vi "gnd_without 3d.vi"() -> ()   [LabVIEW 2015]
doc: "This example performs writes and reads on a serial port, as directed by the user. You can press the Write and Read buttons, and change the Read Count, while the example is running.\n\nThe parameters set for the serial port must match the parameters of the connected instrument or device. In this example, the Read Count parameter specifies the number of bytes that the serial port reads. If there were more bytes at the port than the specified number, those bytes would not be read. If there were less bytes at the port than the specified number, you would receive a timeout error.\n\nThis example expands upon the flow control options for XON and XOFF, allowing the user to choose those control characters. Also, the user can enable or disable a termination character. Some devices require a termination character in order to identify the end of command strings. Some devices send a termination character to signify the end of data to be read. This example shows how you can end the Read operation once a termination character is detected in the buffer and/or append a termination character at the end of the Write data."
uses:
  Program Files/National Instruments/LabVIEW 2015/examples/Instrument IO/Serial/support/Serial - Settings.ctl
  <vilib>/Instr/_visa.llb/VISA Configure Serial Port (Instr).vi
panel:
  out "Euler Angle Chart":cluster{"Pitch":sgl, "Roll":sgl, "Yaw":sgl}(graph)
  out "Servo Angle Chart":T1(graph)
  in  "Period":u32=50
  out "Frequency":dbl
  out "Right_Servo_Angle":string
  out "Left_Servo_Angle":string
  out "Altitude":string
  out "Latitude":string
  in  "Current Satellite Position":refnum<k7>(container)
  out "String":string
  out "current time":timestamp format="%<%H:%M:%S%2u>T"
  out "Longditude":string
  out "Yaw":string
  out "Roll":string
  out "Pitch":string
  out "Start Byte":string
  out "From":string
  in  "Read Count":u32=1000
  in  "Stop Button":bool
  out "length":i32
  out "substring":string
  in  "Start Byte":string
  out "Data Log":string
  in  "Serial Settings":T2={"baud rate"=9600, "data bits"=8, "parity"=enum."None", "stop bits"=10, "flow control"=0} {"flow control" items=["None"=0, "XON/XOFF"=1, "RTS/CTS"=2, "DTR/DSR"=4]; "stop bits" items=["1.0"=10, "1.5"=15, "2.0"=20]; "data bits" min=5 max=8 step=1; "baud rate" items=["75"=75, "110"=110, "134"=134, "150"=150, "300"=300, "600"=600, "1200"=1200, "1800"=1800, "2400"=2400, "4800"=4800, "7200"=7200, "9600"=9600, "14400"=14400, "19200"=19200, "28800"=28800, "38400"=38400, "56000"=56000, "57600"=57600, "115200"=115200, "128000"=128000, "230400"=230400]}
  in  "VISA resource name":refnum<visa-resource-name>="COM1"
  # "2016 SNUSAT CANSAT Competition\nGround Station"
  # "Serial Port Setting"
  # "Serial Read Setting"
  # "Satellite Attitude\n(Euler Angle)"
  # "GPS Position"
  # "Frequency Set (f = 1 / T)"
  # "Servo Angle State"
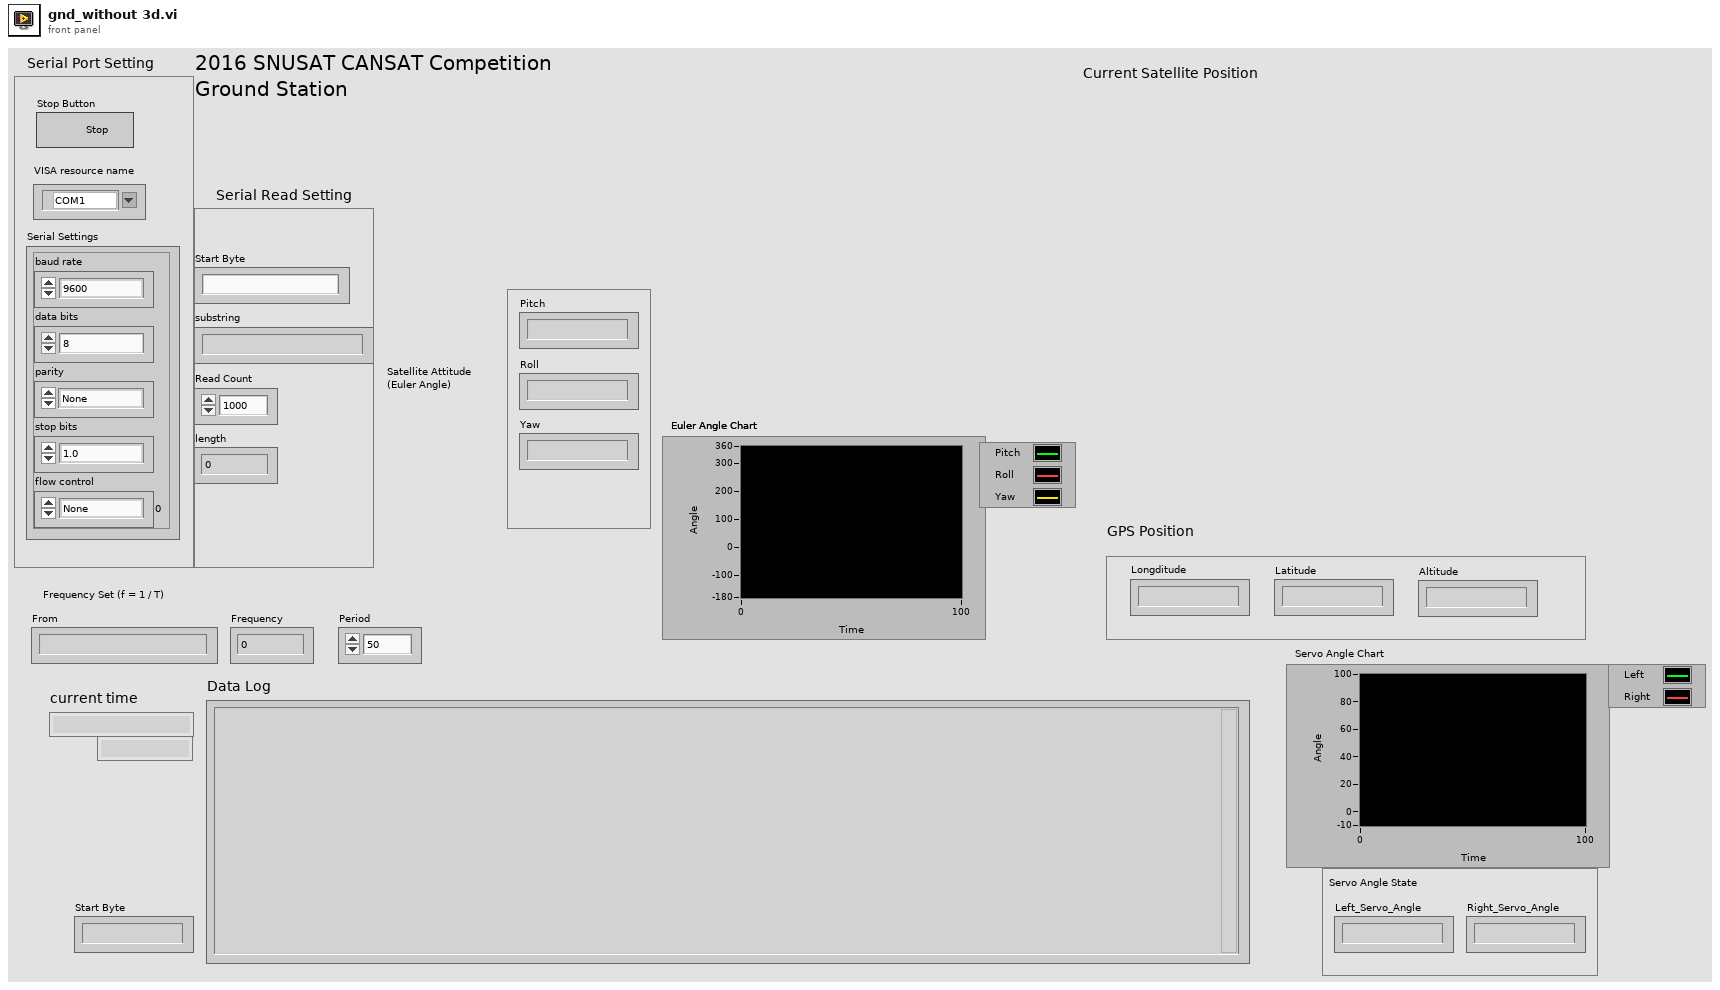
[diagram p1: front panel]
types:
  T1 = cluster{"Left_Servo_Angle":sgl, "Right_Servo_Angle":sgl}
  T2 = typedef "Serial - Settings.ctl" = cluster{"baud rate":u32, "data bits":u16, "parity":enum16{"None", "Odd", "Even", "Mark", "Space"}, "stop bits":u16, "flow control":u16}
  T3 = cluster{"Pitch":string, "Roll":string, "Yaw":string}
  T4 = cluster{"Left_Servo_Angle":string, "Right_Servo_Angle":string}
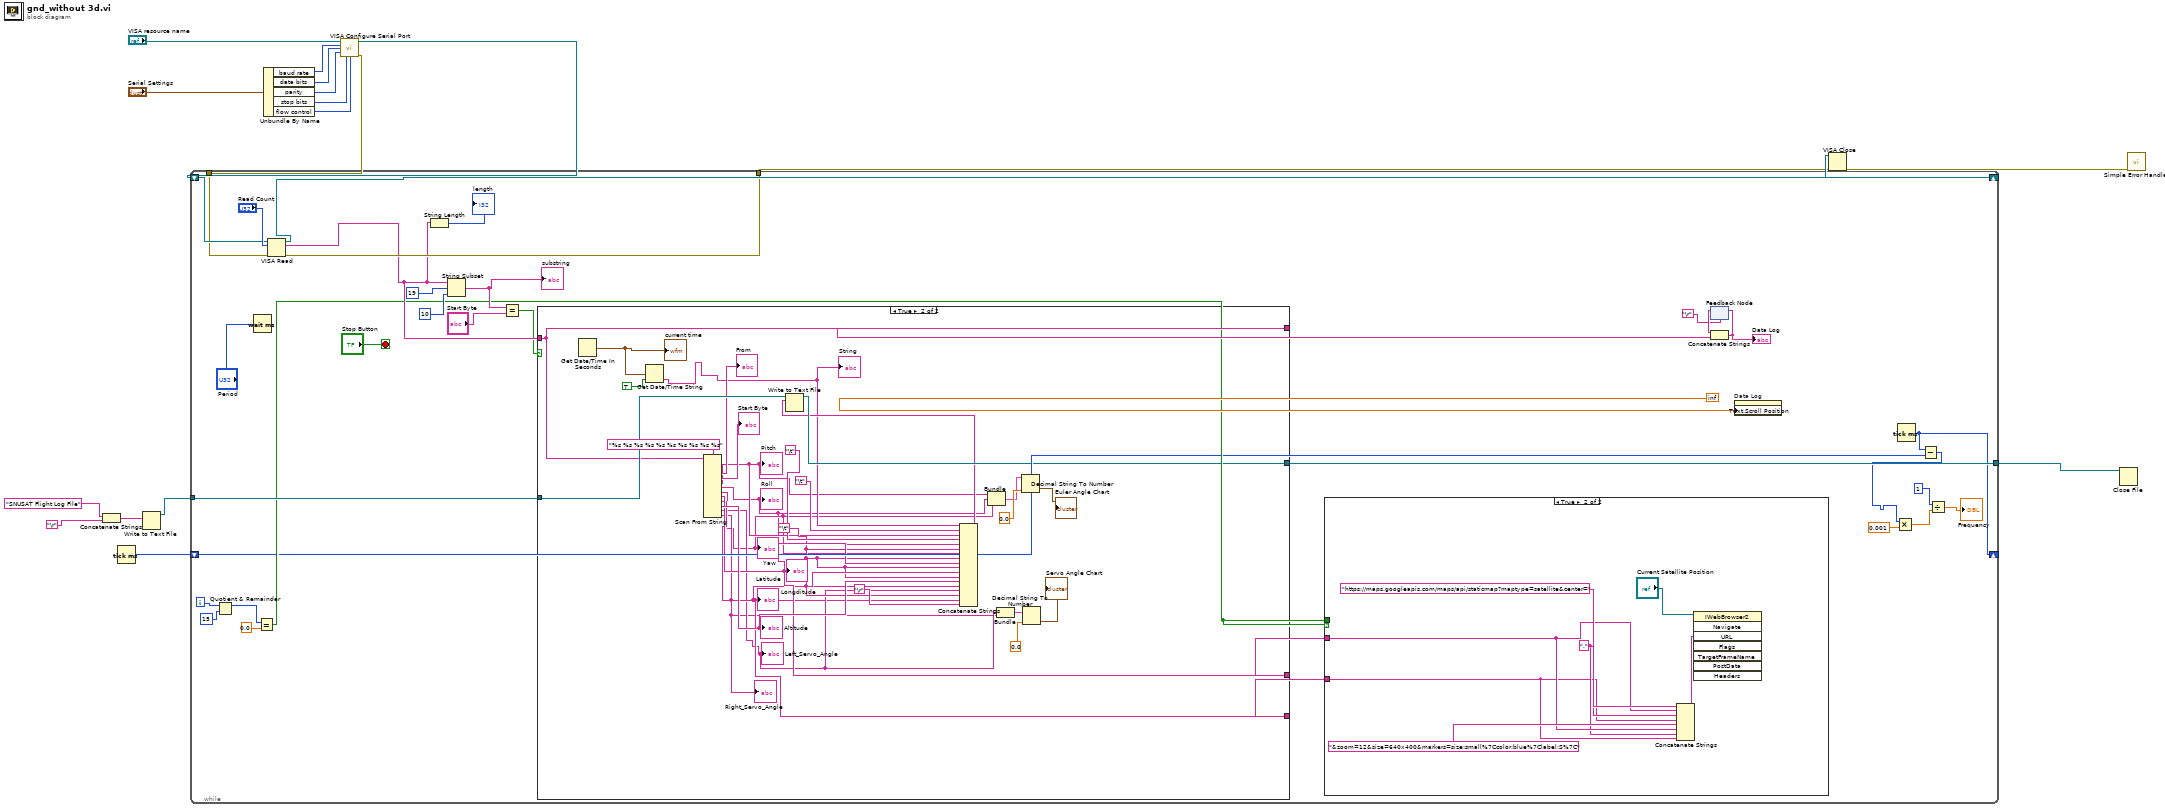
[diagram p0: block diagram]
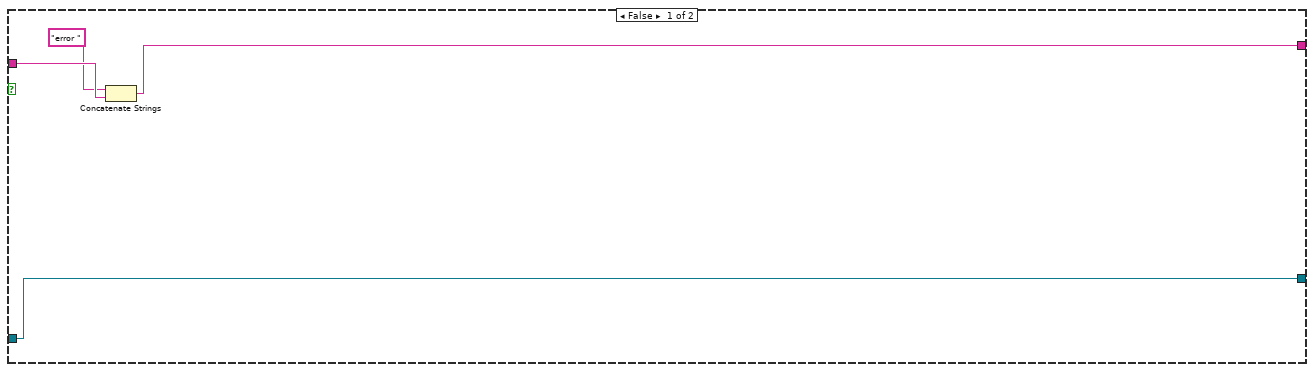
[diagram p3: hidden frame]
diagram:
  n1 = Concatenate Strings("SNUSAT Flight Log File", "\r") -> (w2:string)
  n2 = Tick Count (ms)() -> (millisecond timer value=w1:u32)
  n3 = Write to Text File(text=w2) -> (refnum out=w6:refnum<file>)  [unwired: 3 in, 2 out]
  n4 = Unbundle By Name("Serial Settings") -> ("baud rate"=w14:u32, "data bits"=w15:u16, "parity"=w16:enum16{"None", "Odd", "Even", "Mark", "Space"}, "stop bits"=w17:u16, "flow control"=w11:u16)
  n5 = call-poly "VISA Configure Serial Port"("VISA resource name"="VISA resource name", "baud rate (9600)"=w14, "data bits (8)"=w15, "parity (0:none)"=w16, "stop bits (10: 1 bit)"=w17, "flow control (0:none)"=w11) -> ("VISA resource name out"=w8:refnum<visa-resource-name>, "error out"=w7:errorcluster)  [unwired: 4 in, 4 out]
  n6 = while {
    tunnel: w7 -> [w51]
    tunnel: [w49] -> w9
    shift-right: [w50] -> w10
    shift-left: w8 -> [w52]
    tunnel: w6 -> [w36]
    tunnel: [w35] -> w5
    shift-right: [w19] -> _
    shift-left: w1 -> [w21]
    i -> [w32]
    stop <- "Stop Button" stop-if-true
    n7 = Quotient & Remainder(x=w32, y=15) -> (x-y*floor(x/y)=w29:i32)  [unwired: 1 out]
    n8 = Wait (ms)(milliseconds to wait="Period") -> ()  [unwired: 1 out]
    n9 = Equal?(x=w29, y=0.0) -> (x = y?=w26:bool)
    n10 = VISA Read(VISA resource name=w52, byte count="Read Count", error in (no error)=w51) -> (VISA resource name out=w50:refnum<visa-resource-name>, read buffer=w41:string, error out=w49:errorcluster)  [unwired: 1 out]
    n11 = String Length(string=w41) -> (length=→"length":i32)
    n12 = String Subset(string=w41, offset (0)=19, length (rest)=10 ("length (rest)")) -> (substring=w43:string)
    "substring" <- w43
    n13 = Equal?(x=w43, y="Start Byte") -> (x = y?=w33:bool)
    n14 = case shown="True" w33 {
      tunnel: w41 -> [w64 w87]
      tunnel: [w62 w87] -> w40
      tunnel: w36 -> [w61 w92]
      tunnel: [w61 w91] -> w35
      tunnel: [_ w79] -> w28
      tunnel: [_ w78] -> w27
      frame False {
        n15 = Concatenate Strings("error " ("string"), w64) -> (w62:string)
      }
      frame True {
        w76 = "\t"
        n16 = Get Date/Time In Seconds() -> (seconds since 1Jan1904=w83:timestamp)
        "current time" <- w83
        n17 = Get Date/Time String(seconds (now)=w83, want seconds? (F)=TRUE) -> (time string=w81:string)  [unwired: 1 in, 1 out]
        "String" <- w81
        n18 = Scan From String(format string="%s %s %s %s %s %s %s %s %s %s", input string=w87) -> (output 1=→"From":string, output 2=→"Start Byte":string, output 3=w68:string, output 4=w65:string, output 5=w67:string, output 6=w79:string, output 7=w78:string, output 8=w80:string, output 9=w75:string, output 10=w74:string)  [unwired: 12 in, 3 out]
        "Pitch" <- w68
        "Roll" <- w65
        "Yaw" <- w67
        "Longditude" <- w79
        "Latitude" <- w78
        "Altitude" <- w80
        "Left_Servo_Angle" <- w75
        "Right_Servo_Angle" <- w74
        n19 = Concatenate Strings(w81, "\t", w68, "\t", w65, w76, w67, w76, w79, w76, w78, w76, w80, w76, w75, w76, w74, "\r") -> (w85:string)
        n20 = Write to Text File(file (use dialog)=w92, text=w85) -> (refnum out=w91:refnum<file>)  [unwired: 2 in, 2 out]
        n21 = Bundle("Pitch"=w68, "Roll"=w65, "Yaw"=w67) -> (w69:T3)  [unwired: 1 in]
        n22 = Bundle("Left_Servo_Angle"=w75, "Right_Servo_Angle"=w74) -> (w73:T4)  [unwired: 1 in]
        n23 = Decimal String To Number(string=w69, default (0L)=sgl 0.0 ("Length X")) -> (number=→"Euler Angle Chart":cluster{"Pitch":sgl, "Roll":sgl, "Yaw":sgl})  [unwired: 1 in, 1 out]
        n24 = Decimal String To Number(string=w73, default (0L)=sgl 0.0 ("Length X")) -> (number=→"Servo Angle Chart":T1)  [unwired: 1 in, 1 out]
      }
    }
    n25 = case shown="True" w26 {
      tunnel: w26 -> [_ _]
      tunnel: w28 -> [_ w56]
      tunnel: w27 -> [_ w54]
      frame False {
      }
      frame True {
        w55 = ","
        n26 = Concatenate Strings("https://maps.googleapis.com/maps/api/staticmap?maptype=satellite&center=" ("문자열"), w56, w55, w54, "&zoom=12&size=640x400&markers=size:small%7Ccolor:blue%7Clabel:S%7C", w56, w55, w54) -> (w59:string)
        n27 = invoke class="IWebBrowser2" method="Navigate"(reference="Current Satellite Position", "URL"=w59) -> ()  [unwired: 6 in, 8 out]
      }
    }
    n28 = feedback #1("\r") -> (w39:string)
    n29 = Concatenate Strings(w39, w40) -> (w38:string)
    "Data Log" <- w38
    n30 = feedback-in #1(w38) -> ()
    n31 = property on="Data Log" class="Str"("Text.Scroll Position"=inf) -> ()  [unwired: 2 in, 2 out]
    n32 = Tick Count (ms)() -> (millisecond timer value=w19:u32)
    n33 = Subtract(x=w19, y=w21) -> (x-y=w20:u32)
    n34 = Multiply(x=w20, y=0.001) -> (x*y=w23:dbl)
    n35 = Divide(x=1, y=w23) -> (x/y=→"Frequency":dbl)
  }
  n36 = VISA Close(VISA resource name=w10, error in (no error)=w9) -> (error out=w12:errorcluster)
  n37 = Close File(refnum=w5) -> ()  [unwired: 1 in, 2 out]
  n38 = call <vilib>:"Simple Error Handler.vi"("error in (no error)"=w12) -> ()  [unwired: 1 in, 8 out]
